vi "Main power.vi"() -> ()   [LabVIEW 2020]
uses:
  Commande.ctl
  <vilib>/Instr/_visa.llb/VISA Configure Serial Port (Instr).vi
  <instrlib>/Sorensen SG Series/Sorensen SG Series.lvlib
panel:
  in  "Alim":enum32{"Item 0", "Item 1"}(radio)
  out "Voltage level":string
  out "Read V":string
  out "Read I":string
  out "error out":errorcluster
  out "Actual PowerLevel (W)":dbl format="%.3f"
  out "Booléen":bool
  out "status":bool
  out "Actual Current Level (A)":dbl format="%.3f"
  out "Actual Voltage Level (V)":dbl format="%.3f"
  out "Message":string
  in  "U Level":dbl step=0.1
  in  "Power":bool
  in  "I Limit":dbl=100.0
  in  "U limit":dbl=8.0
  in  "STOP":bool
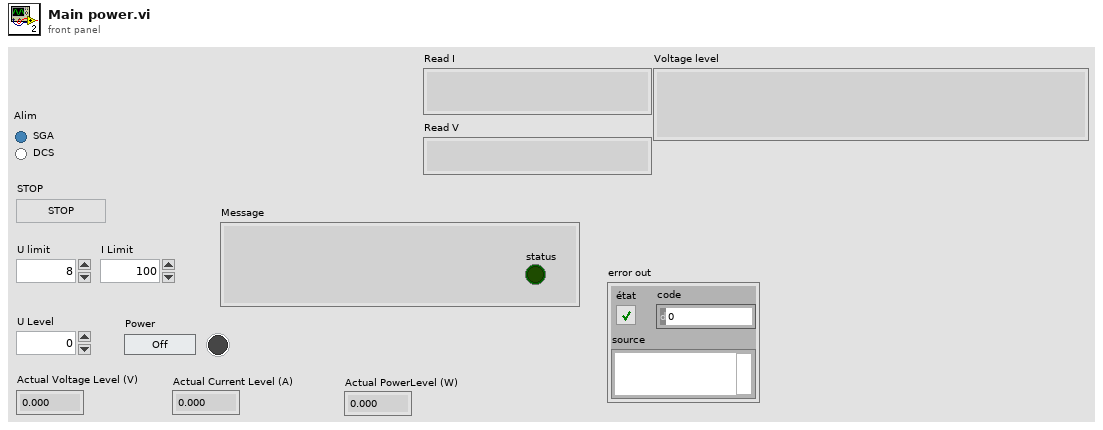
[diagram p1: front panel]
types:
  T1 = typedef "Commande.ctl" = enum16{"Power ON/OFF", "WaitForEvent", "Limit U&I", "Send ui", "Send U", "Meas", "Stop", "Init"}
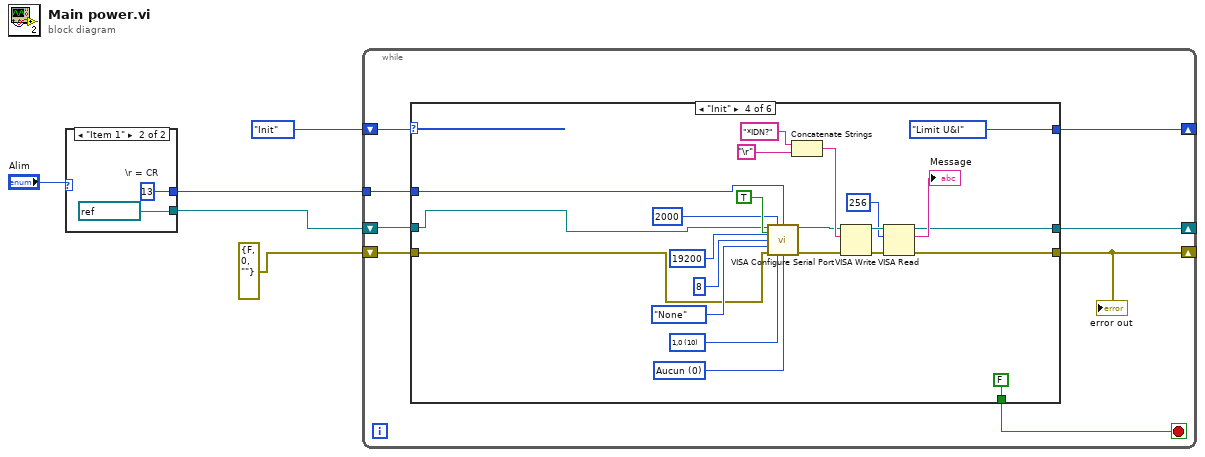
[diagram p0: block diagram]
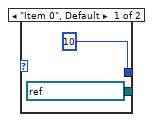
[diagram p2: hidden frame]
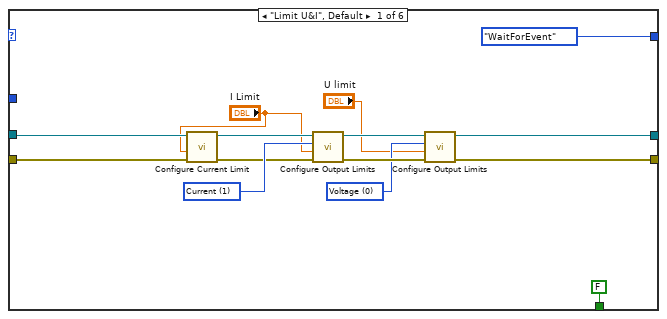
[diagram p3: hidden frame]
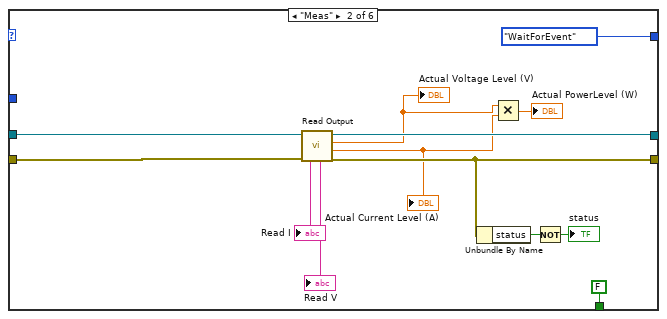
[diagram p4: hidden frame]
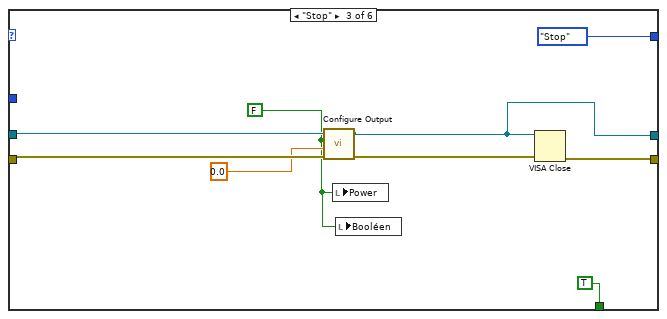
[diagram p5: hidden frame]
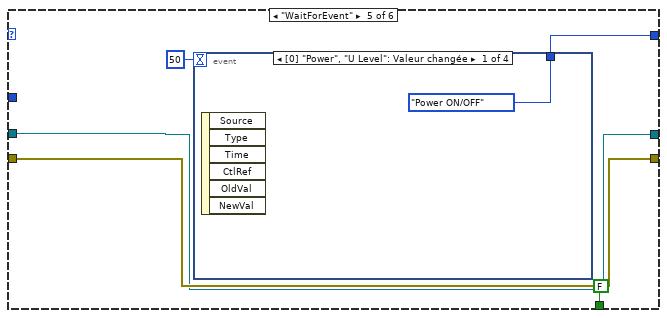
[diagram p6: hidden frame]
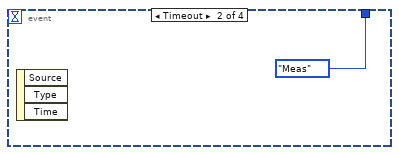
[diagram p7: hidden frame]
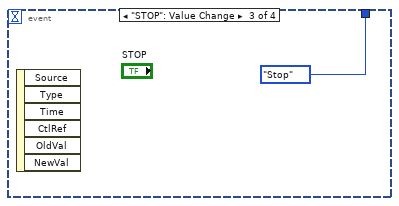
[diagram p8: hidden frame]
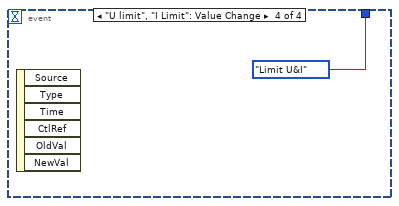
[diagram p9: hidden frame]
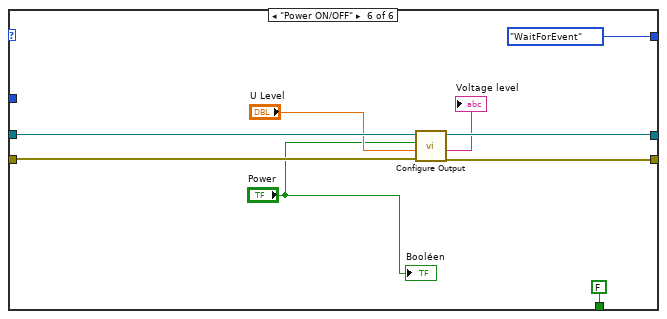
[diagram p10: hidden frame]
diagram:
  n1 = case shown="\"Item 1\"" "Alim" {
    tunnel: [u8 10 ("\\n = LF") w9] -> w3
    tunnel: [refnum<visa-resource-name> "ASRL5::INSTR" ("VISA resource name") refnum<visa-resource-name> "COM4" ("VISA resource name")] -> w2
    frame "Item 0", Default {
    }
    frame "Item 1" {
      w9 = u8 13  # \r = CR
    }
  }
  n2 = while {
    shift-right: [w15] -> _
    shift-left: Commande."Init" -> [w17]
    shift-right: [w14] -> _
    shift-left: w2 -> [w12]
    shift-right: [w13] -> _
    shift-left: errorcluster {"status"=FALSE, "code"=0, "source"=""} ("error in (no error)") -> [w11]
    tunnel: w3 -> [w10]
    stop <- w16 stop-if-true
    n3 = case shown="\"Init\"" w17 {
      tunnel: [FALSE FALSE TRUE FALSE FALSE FALSE] -> w16
      tunnel: [Commande."WaitForEvent" Commande."WaitForEvent" Commande."Stop" Commande."Limit U&I" w81 Commande."WaitForEvent"] -> w15
      tunnel: [w24 w44 w47 w57 w78 w91] -> w14
      tunnel: [w23 w41 w51 w56 w79 w90] -> w13
      tunnel: w12 -> [w22 w33 w50 w54 w78 w94]
      tunnel: w11 -> [w21 w32 w49 w62 w79 w93]
      tunnel: w10 -> [_ _ _ w55 _ _]
      frame "Limit U&I", Default {
        w26 = u16 0 items=["Voltage", "Current"] ("Measurement Type (0:Voltage)")
        w29 = u16 1 items=["Voltage", "Current"] ("Measurement Type (0:Voltage)")
        n4 = call "Configure Current Limit.vi"("error in (no error)"=w21, "Current Limit (0.00 A)"="I Limit", "VISA resource name"=w22) -> ("error out"=w19:errorcluster, "VISA resource name out"=w20:refnum<visa-resource-name>)  [unwired: 6 in, 1 out]
        n5 = call <instrlib>:"Configure Output Limits.vi"("error in (no error)"=w19, "Soft Limit (0.00)"="I Limit", "Measurement Type (0:Voltage)"=w29, "VISA resource name"=w20) -> ("error out"=w27:errorcluster, "VISA resource name out"=w28:refnum<visa-resource-name>)  [unwired: 6 in]
        n6 = call <instrlib>:"Configure Output Limits.vi"("error in (no error)"=w27, "Soft Limit (0.00)"="U limit", "Measurement Type (0:Voltage)"=w26, "VISA resource name"=w28) -> ("error out"=w23:errorcluster, "VISA resource name out"=w24:refnum<visa-resource-name>)  [unwired: 6 in]
      }
      frame "Meas" {
        n7 = call "Read Output.vi"("error in (no error)"=w32, "VISA resource name"=w33) -> ("error out"=w41:errorcluster, "Actual Current Level (A)"=w37:dbl, "Actual Voltage Level (V)"=w38:dbl, "VISA resource name out"=w44:refnum<visa-resource-name>, "Read V"=→"Read V":string, "Read I"=→"Read I":string)  [unwired: 4 in]
        "Actual Voltage Level (V)" <- w38
        "Actual Current Level (A)" <- w37
        n8 = Unbundle By Name(w41) -> ("status"=w40:bool)
        n9 = Multiply(x=w38, y=w37) -> (x*y=→"Actual PowerLevel (W)":dbl)
        n10 = Not(x=w40) -> (.not. x?=→"status":bool)
      }
      frame "Stop" {
        w45 = FALSE ("Enable Output (T: Enable)")
        n11 = call "Configure Output.vi"("error in (no error)"=w49, "Voltage Level (0.00 V)"=0.0, "Enable Output (T: Enable)"=w45, "VISA resource name"=w50) -> ("error out"=w46:errorcluster, "VISA resource name out"=w47:refnum<visa-resource-name>)  [unwired: 5 in, 1 out]
        n12 = local write "Power"(w45) -> ()
        n13 = local write "Booléen"(w45) -> ()
        n14 = VISA Close(VISA resource name=w47, error in (no error)=w46) -> (error out=w51:errorcluster)
      }
      frame "Init" {
        w72 = u16 10 items=["1,0"=10, "1,5"=15, "2,0"=20] ("stop bits (10: 1 bit)")
        w71 = u16 0 items=["Aucun", "XON/XOFF", "RTS/CTS", "XON/XOFF & RTS/CTS", "DTR/DSR", "XON/XOFF & DTR/DSR"] ("flow control (0:none)")
        n15 = call-poly "VISA Configure Serial Port"("VISA resource name"=w54, "timeout (10sec)"=u32 2000, "termination char\n(0xA = '\\n' = LF)"=w55, "Enable Termination\nChar (T)"=TRUE ("Enable Termination\nChar (T)"), "baud rate (9600)"=u32 19200, "data bits (8)"=u16 8, "parity (0:none)"=enum16{"None", "Odd", "Even", "Mark", "Space"}."None", "error in (no error)"=w62, "stop bits (10: 1 bit)"=w72, "flow control (0:none)"=w71) -> ("VISA resource name out"=w64:refnum<visa-resource-name>, "error out"=w63:errorcluster)  [unwired: 4 in]
        n16 = Concatenate Strings("*IDN?", "\r") -> (w70:string)
        n17 = VISA Write(VISA resource name=w64, write buffer=w70, error in (no error)=w63) -> (VISA resource name out=w68:refnum<visa-resource-name>, error out=w69:errorcluster)  [unwired: 1 out]
        n18 = VISA Read(VISA resource name=w68, byte count=u32 256 ("nombre d'octets"), error in (no error)=w69) -> (VISA resource name out=w57:refnum<visa-resource-name>, read buffer=→"Message":string, error out=w56:errorcluster)  [unwired: 1 out]
      }
      frame "WaitForEvent" {
        n19 = event shown="[0] \"Power\", \"U Level\": Valeur changée" {
          selector: _ -> [_ _ _ _]
          dyn-events: _ -> [_ _ _ _]
          timeout: 50 -> [_ _ _ _]
          tunnel: [Commande."Power ON/OFF" Commande."Meas" Commande."Stop" Commande."Limit U&I"] -> w81
          event "Power", "U Level": Value Change {
            n20 = event-data() -> ()  [unwired: 1 in, 6 out]
          }
          event Timeout {
            n21 = event-data() -> ()  [unwired: 1 in, 3 out]
          }
          event "STOP": Value Change {
            n22 = event-data() -> ()  [unwired: 1 in, 6 out]
          }
          event "U limit", "I Limit": Value Change {
            n23 = event-data() -> ()  [unwired: 1 in, 6 out]
          }
        }
      }
      frame "Power ON/OFF" {
        n24 = call "Configure Output.vi"("error in (no error)"=w93, "Voltage Level (0.00 V)"="U Level", "Enable Output (T: Enable)"="Power", "VISA resource name"=w94) -> ("error out"=w90:errorcluster, "Voltage level"=→"Voltage level":string, "VISA resource name out"=w91:refnum<visa-resource-name>)  [unwired: 5 in]
        "Booléen" <- "Power"
      }
    }
    "error out" <- w13
  }
